vi "Screen_Test.vi"() -> ()   [LabVIEW 2011]
uses:
  030 - EVENTS/EnumFgvEventCommand.ctl
  090 - ERRORS/Ctrls/enumLogAndView.ctl
  SubVis/Ctrls/EnumLockUnlockScreen.ctl
  enumScreen.ctl
  100_PROCESS/SubVis/Enum_HideShow_Process.ctl
  03 - POPUPS/Popup_ShowHideProcess.ctl
  100_PROCESS/SubVis/EnumFgvReferenceProcess.ctl
  100_PROCESS/EnumProcess.ctl
  090 - ERRORS/Ctrls/EnumErrors.ctl
  SubVis/Ctrls/EnumStartStopProgressBar.ctl
  SubVis/Ctrls/EnumEnableDisableClose.ctl
panel:
  out "Process":T1[](array[typedef])
  in  "Window_State":T3(ring)=enum."Standard"
  in  "BoutonSetWindowState":bool
  in  "Hide / Show front panel":T2
  in  "BoutonShowHide":bool
  in  "Bouton menu principal":bool
  in  "Clear message":bool
  in  "Send Error X 100":bool
  in  "Load previous screen":bool
  in  "message":string
  in  "ErrorCode":T4
  in  "Send Error":bool
  in  "Load SCREEN":T5=enum."LOG"
  in  "Close application":bool
  in  "LockUnlock":bool
  in  "Progress bar value":u8(slide) max=100 scale=0.0..100.0
  in  "Automatic progress bar on ?":T6=enum."Stop progress bar"
  in  "Enable close ?":T7
  # "Ecran de test"
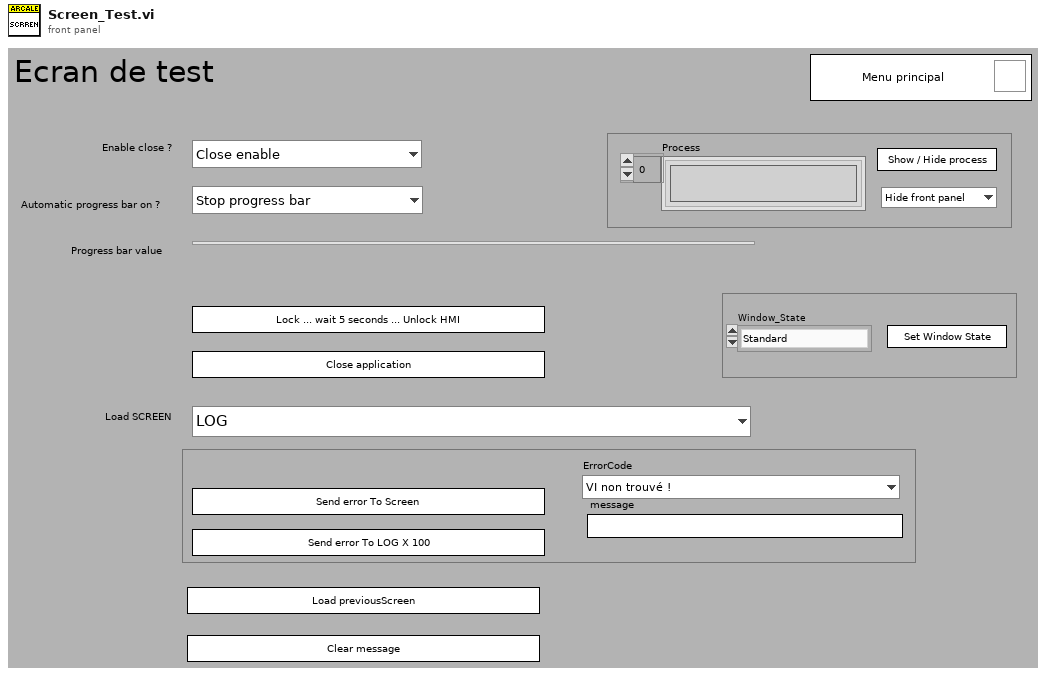
[diagram p1: front panel]
types:
  T1 = typedef "Popup_ShowHideProcess.ctl" = cluster{"Path":path, "VI Name":string, "Hide / Show":T2}
  T2 = typedef "Enum_HideShow_Process.ctl" = enum16{"Hide front panel", "Show front panel"}
  T3 = enum32{"Invalid", "Standard", "Closed", "Hidden", "Minimized", "Maximized"}
  T4 = typedef "EnumErrors.ctl" = enum16{"VI non trouvé !", "Clé non trouvée", "Timeout", "Le VI tourne déjà", "Erreur de séparateur décimal", "Référence non trouvée"}
  T5 = typedef "enumScreen.ctl" = enum16{"Test screen", "Ecran principal", "LOG", "Setup", "Popup : About", "Popup : View last message", "Popup : WebBrowser help", "Traduction", "Popup : DEBUG Process"}
  T6 = typedef "EnumStartStopProgressBar.ctl" = enum16{"Start progress bar", "Stop progress bar"}
  T7 = typedef "EnumEnableDisableClose.ctl" = enum16{"Close enable", "Close disable"}
  T8 = typedef "EnumProcess.ctl" = enum16{"Message handler", "Template"}
  T9 = typedef "EnumFgvReferenceProcess.ctl" = enum16{"Init", "Get", "Add Reference", "Close References"}
  T10 = typedef "enumLogAndView.ctl" = enum16{"Log only", "Log and view"}
  T11 = typedef "EnumFgvEventCommand.ctl" = enum16{"Setup", "Cleanup", "Get"}
  T12 = typedef "EnumLockUnlockScreen.ctl" = enum16{"Lock screen", "Unlock screen"}
  T13 = typedef "ToScreensCommand.ctl" = enum16{"Stop screen", "Stop all screens"}
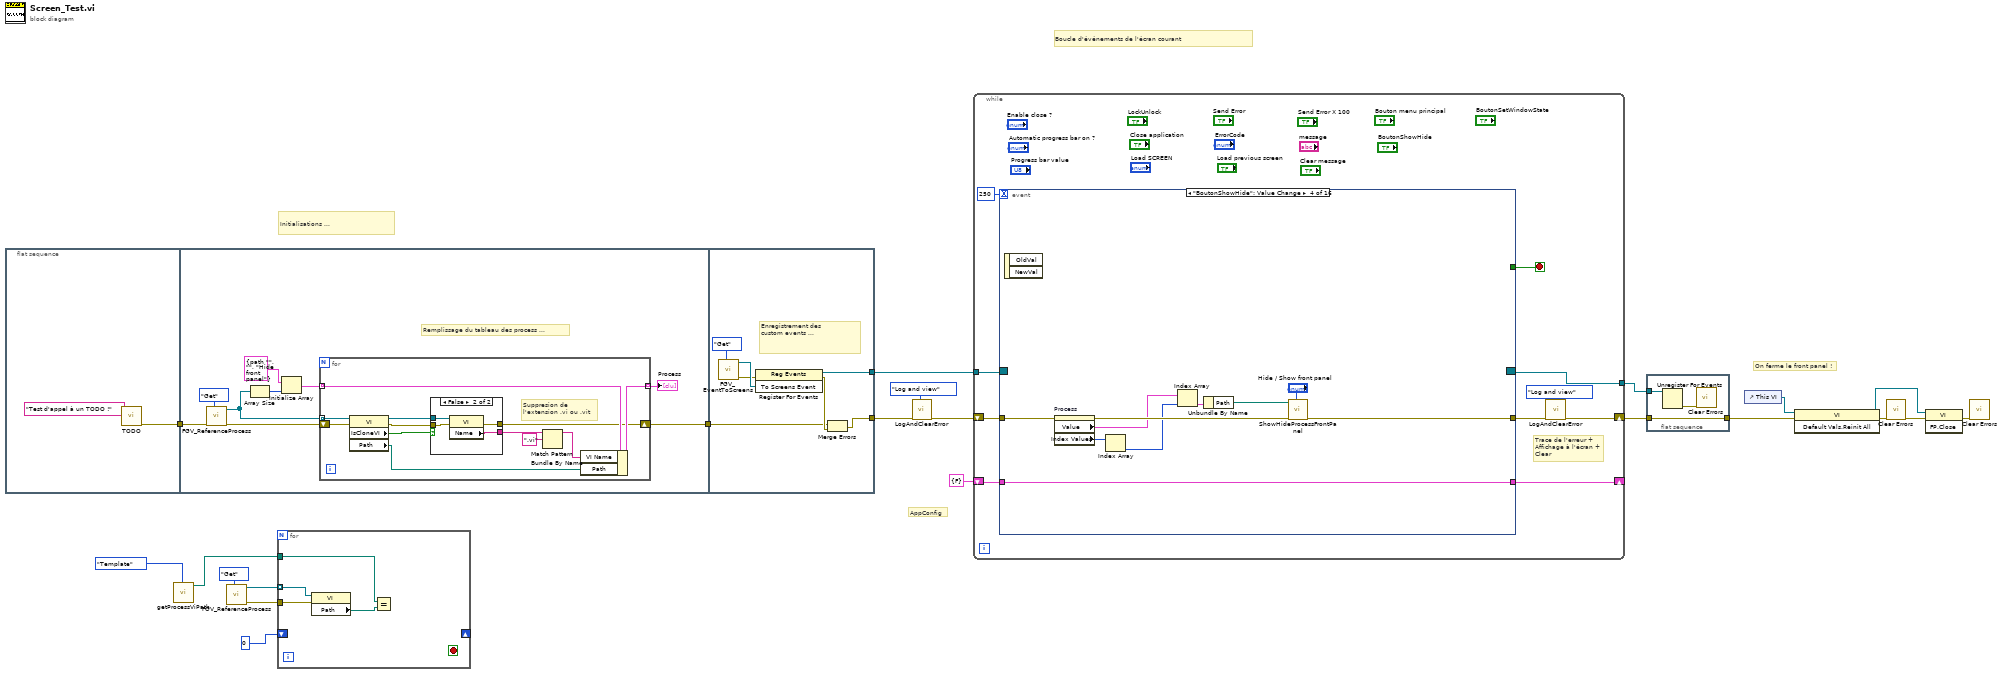
[diagram p0: block diagram]
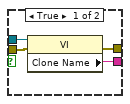
[diagram p2: hidden frame]
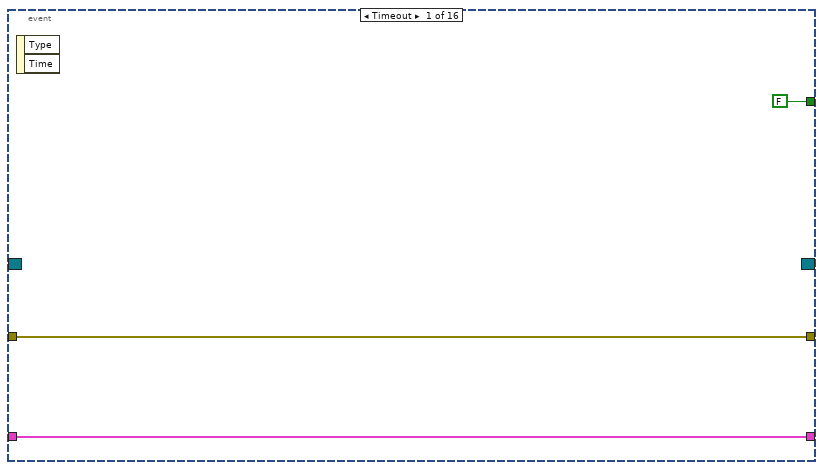
[diagram p3: hidden frame]
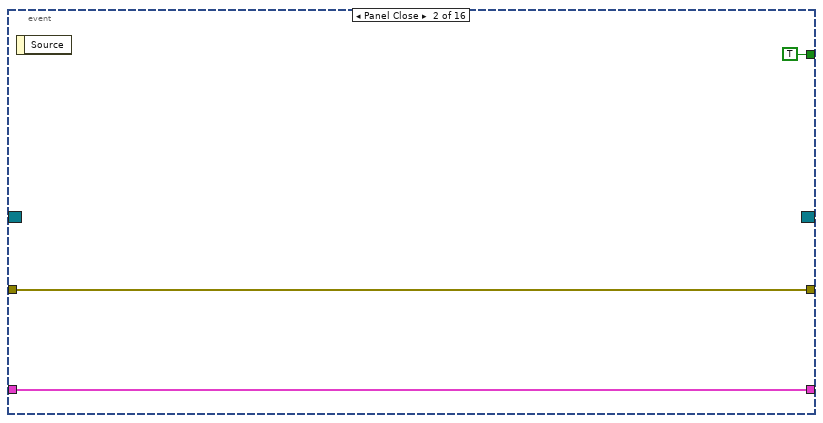
[diagram p4: hidden frame]
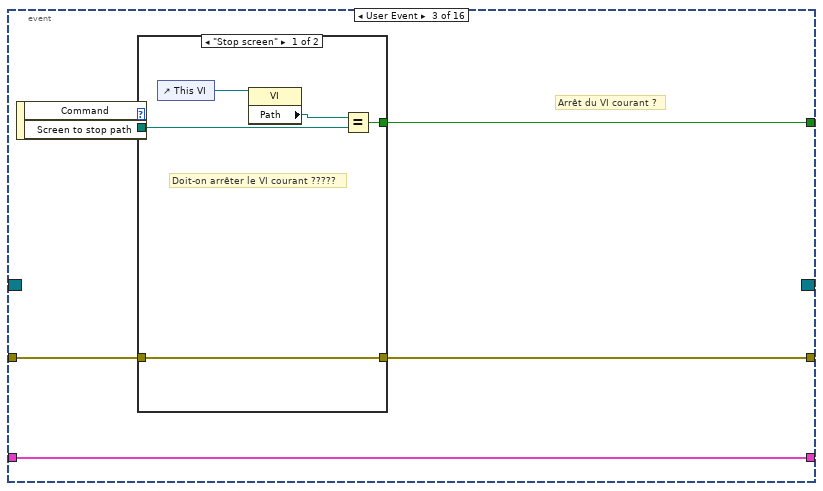
[diagram p5: hidden frame]
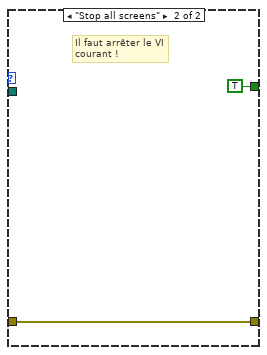
[diagram p6: hidden frame]
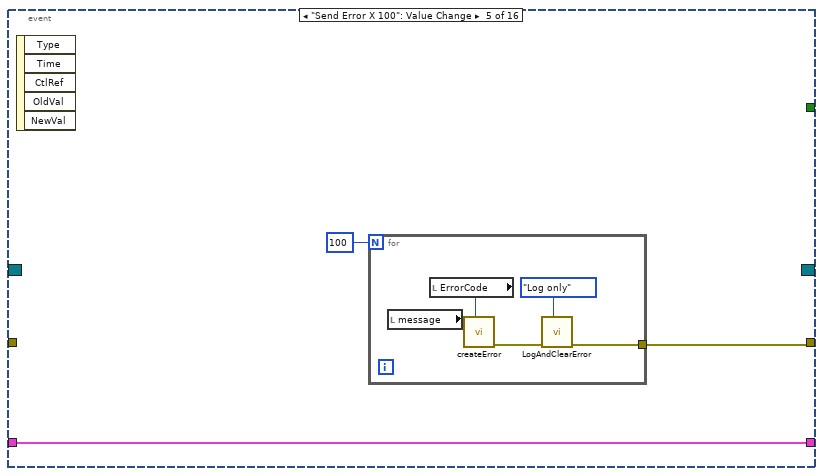
[diagram p7: hidden frame]
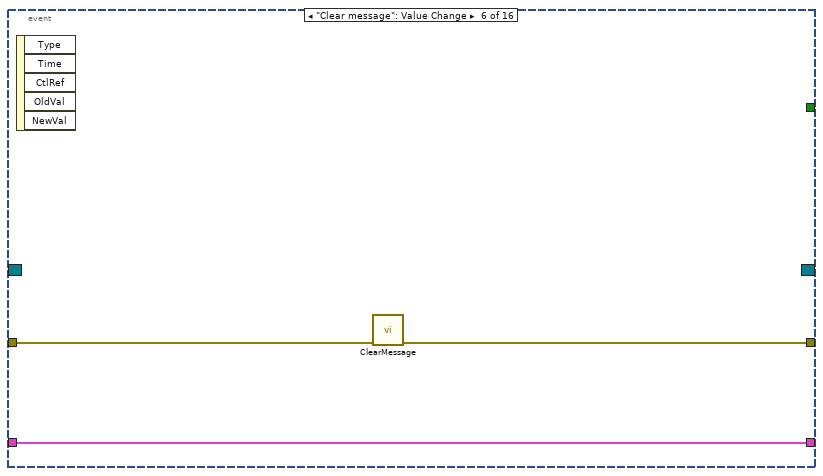
[diagram p8: hidden frame]
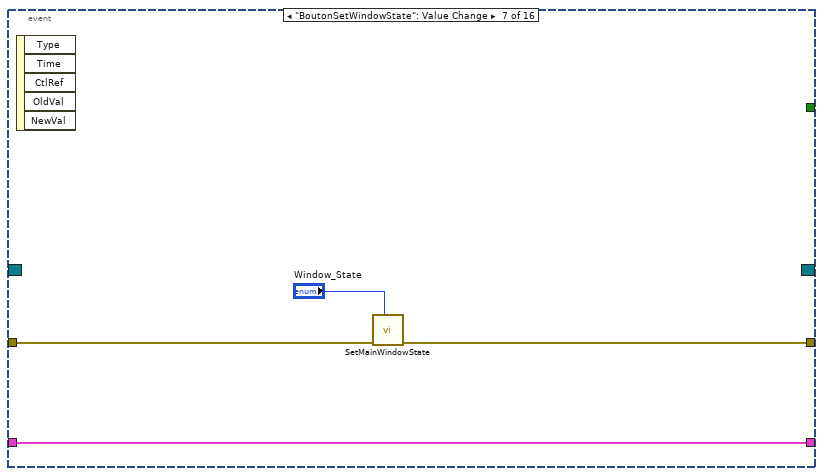
[diagram p9: hidden frame]
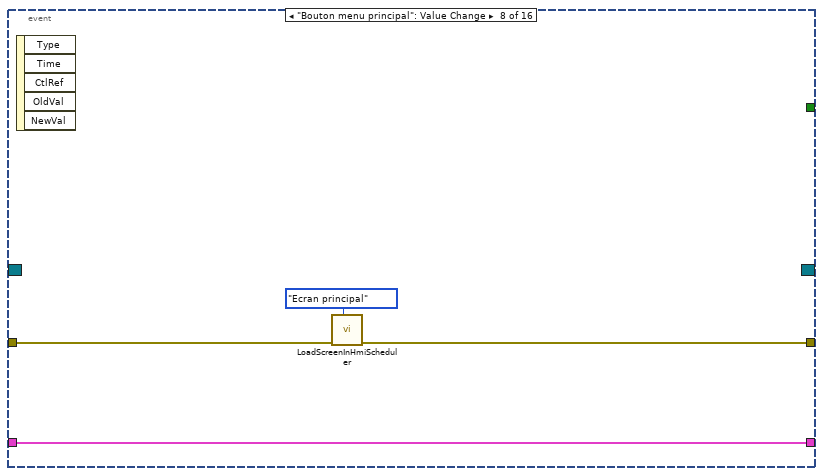
[diagram p10: hidden frame]
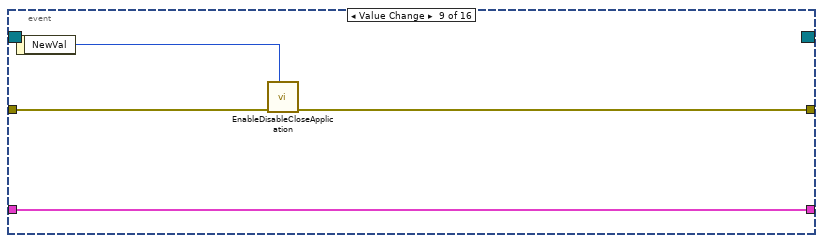
[diagram p11: hidden frame]
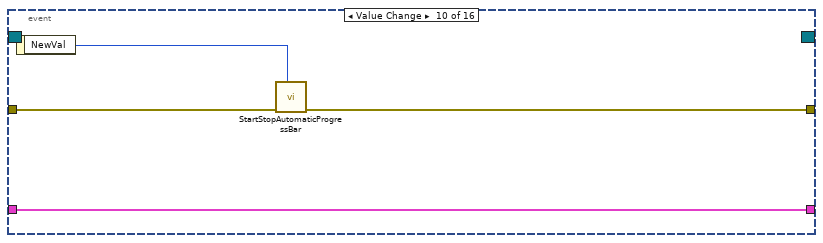
[diagram p12: hidden frame]
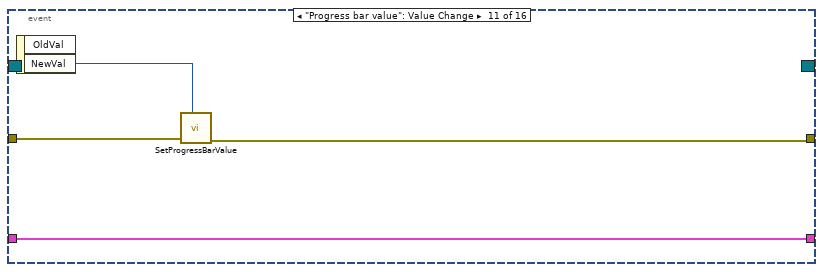
[diagram p13: hidden frame]
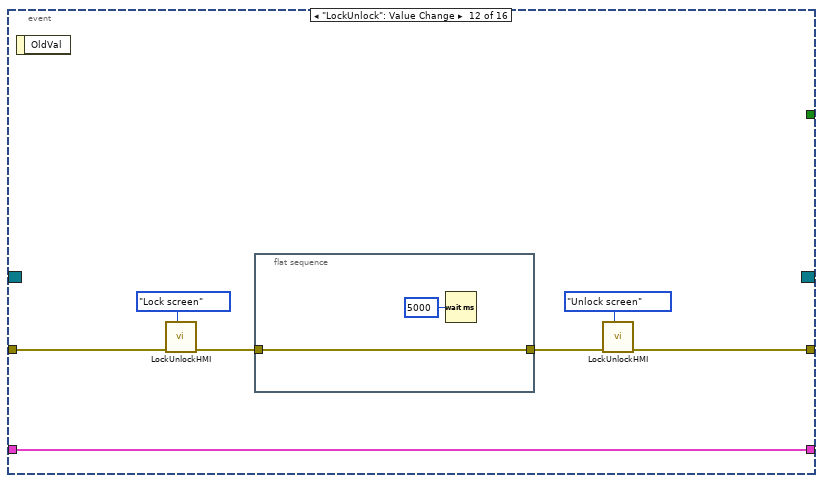
[diagram p14: hidden frame]
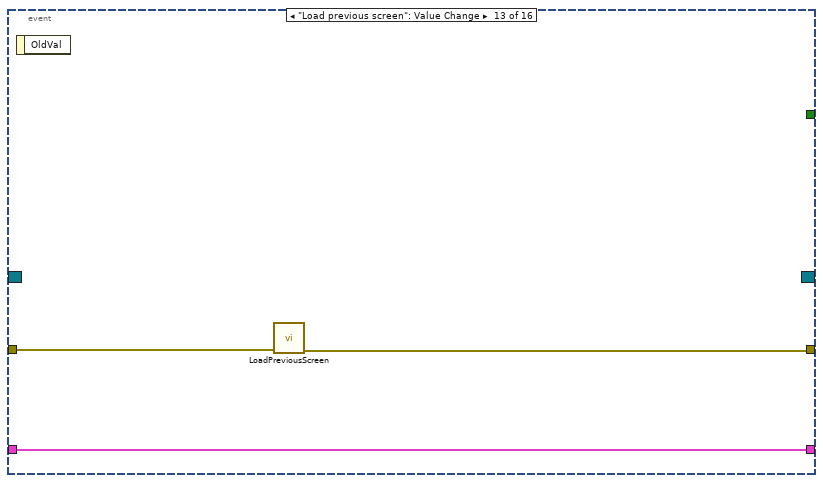
[diagram p15: hidden frame]
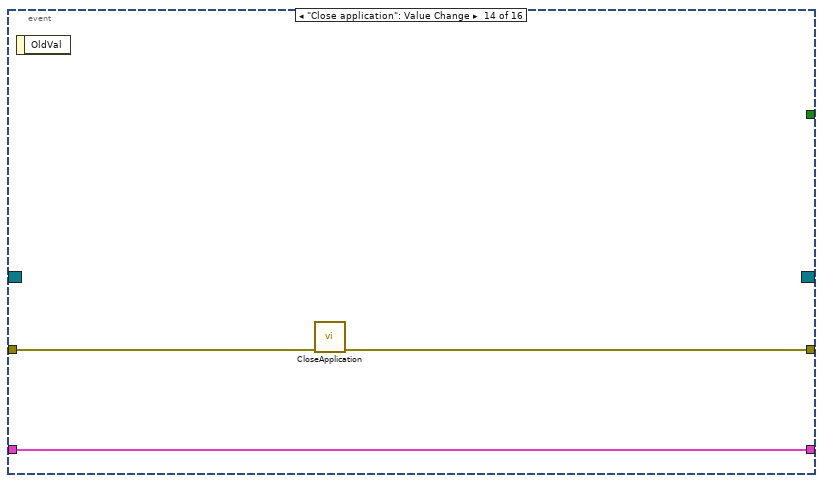
[diagram p16: hidden frame]
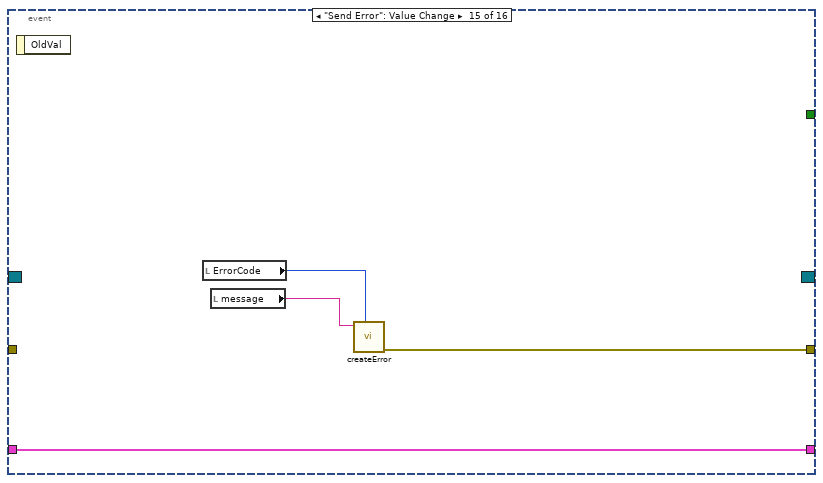
[diagram p17: hidden frame]
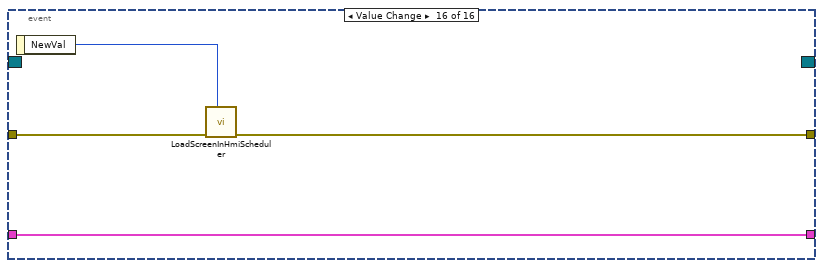
[diagram p18: hidden frame]
diagram:
  # "AppConfig"
  # "Initialisations ..."
  # "On ferme le front panel !"
  # "Boucle d'événements de l'écran courant"
  n1 = flat-sequence {
    tunnel: [w22] -> w8
    tunnel: w8 -> [w27]
    tunnel: [w26] -> w7
    tunnel: w7 -> [w54]
    tunnel: [w55] -> w17
    tunnel: [w53] -> w14
    frame #0 {
      n2 = call "TODO.vi"("Message"="Test d'appel à un TODO !") -> ("error out"=w22:errorcluster)  [unwired: 10 in]
    }
    frame #1 {
      # "Remplissage du tableau des process ..."
      n3 = call "FGV_ReferenceProcess.vi"("Commande"=EnumFgvReferenceProcess."Get", "error in (no error)"=w27) -> ("error out"=w29:errorcluster, "ProcessReferences"=w28:refnum<vi>[])  [unwired: 8 in]
      n4 = Array Size(array=w28) -> (size(s)=w31:i32)
      n5 = Initialize Array(T1 {"Path"=path "", "VI Name"="", "Hide / Show"=enum."Hide front panel"}, w31) -> (w30:T1[])
      n6 = for {
        tunnel: [w44] -> w25 mode=indexing
        tunnel: w28 -> [w41] mode=indexing
        tunnel: w30 -> [w43] mode=indexing
        shift-right: [w36] -> w26
        shift-left: w29 -> [w42]
        # "Suppresion de l'extension .vi ou .vit"
        n7 = property class="VI"(reference=w41, error in=w42) -> (reference out=w38:refnum<vi>, error out=w37:errorcluster, "IsCloneVI"=w39:bool, "Path"=w40:path)
        n8 = case shown="False" w39 {
          tunnel: w38 -> [w48 w52]
          tunnel: w37 -> [w47 w51]
          tunnel: [w46 w50] -> w36
          tunnel: [w45 w49] -> w34
          frame True {
            n9 = property class="VI"(reference=w48, error in=w47) -> (error out=w46:errorcluster, "Clone Name"=w45:string)  [unwired: 1 out]
          }
          frame False {
            n10 = property class="VI"(reference=w52, error in=w51) -> (error out=w50:errorcluster, "Name"=w49:string)  [unwired: 1 out]
          }
        }
        n11 = Match Pattern(string=w34, regular expression=".vi") -> (before substring=w33:string)  [unwired: 1 in, 3 out]
        n12 = Bundle By Name(cluster=w43, "VI Name"=w33, "Path"=w40) -> (w44:T1)
      }
      "Process" <- w25
    }
    frame #2 {
      # "Enregistrement des\ncustom events ..."
      n13 = call "FGV_EventToScreens.vi"("Command"=EnumFgvEventCommand."Get") -> ("error out"=w57:errorcluster, "To Screens Event"=w58:refnum<user-event>)  [unwired: 9 in]
      n14 = register-events(error in=w57, w58) -> (reference out=w55:refnum<event-registration>, error out=w59:errorcluster)  [unwired: 1 in]
      n15 = Merge Errors(w54, w59) -> (w53:errorcluster)
    }
  }
  n16 = call "getProcessViPath.vi"("Enum Screen"=EnumProcess."Template" ("Process")) -> ("Path"=w2:path)  [unwired: 9 in, 1 out]
  n17 = call "FGV_ReferenceProcess.vi"("Commande"=EnumFgvReferenceProcess."Get") -> ("error out"=w4:errorcluster, "ProcessReferences"=w5:refnum<vi>[])  [unwired: 9 in]
  n18 = for {
    tunnel: w5 -> [w63] mode=indexing
    tunnel: w4 -> [w62]
    tunnel: w2 -> [w60]
    shift-right: _ -> [_]
    shift-left: 0 -> [_]
    stop <- _ stop-if-true
    n19 = property class="VI"(reference=w63, error in=w62) -> ("Path"=w61:path)  [unwired: 2 out]
    n20 = Equal?(x=w60, y=w61) -> ()  [unwired: 1 out]
  }
  n21 = call "LogAndClearError.vi"("Log and view ?"=enumLogAndView."Log and view", "error in (no error)"=w14) -> ("error out"=w15:errorcluster)  [unwired: 9 in]
  n22 = while {
    tunnel: w17 -> [w73]
    shift-right: [w67] -> w20
    shift-left: w15 -> [w72]
    tunnel: [w71] -> w21
    shift-right: [w68] -> _
    shift-left: cluster{"Boolean":bool} {"Boolean"=FALSE} ("appContext") -> [w69]
    stop <- w70 stop-if-true
    # "Trace de l'erreur +\nAffichage à l'écran +\nClear"
    n23 = event shown="[3] \"BoutonShowHide\": Value Change" {
      selector: w73 -> [_ _ _ _ _ _ _ _ _ _ _ _ _ _ _ _]
      dyn-events: [_ _ _ _ _ _ _ _ _ _ _ _ _ _ _ _] -> w71
      timeout: 250 -> [_ _ _ _ _ _ _ _ _ _ _ _ _ _ _ _]
      tunnel: w72 -> [w76 w79 w84 w99 _ w113 w117 w120 w124 w129 w133 w140 w145 w148 _ w156]
      tunnel: [w76 w79 w83 w102 w105 w112 w116 w119 w123 w128 w132 w136 w144 w147 w150 w154] -> w66
      tunnel: [FALSE TRUE w81 _ _ _ _ _ _ _ _ _ _ _ _ _] -> w70
      tunnel: w69 -> [w74 w78 w80 w101 w103 w111 w115 w121 w125 w127 w131 w139 w143 w146 w152 w153]
      tunnel: [w74 w78 w80 w101 w103 w111 w115 w121 w125 w127 w131 w139 w143 w146 w152 w153] -> w68
      event Timeout {
        n24 = event-data() -> ()  [unwired: 1 in, 2 out]
      }
      event Panel Close {
        n25 = event-data() -> ()  [unwired: 1 in, 1 out]
      }
      event User Event {
        # "Arrêt du VI courant ?"
        n26 = event-data() -> ("Command"=w85:T13, "Screen to stop path"=w82:path)  [unwired: 1 in]
        n27 = case shown="\"Stop screen\"" w85 {
          tunnel: w84 -> [w90 w91]
          tunnel: [w90 w91] -> w83
          tunnel: w82 -> [w87 _]
          tunnel: [w86 TRUE] -> w81
          frame "Stop screen" {
            # "Doit-on arrêter le VI courant ?????"
            n28 = control-ref of="This VI"() -> (w89:refnum<vi>)
            n29 = property class="VI"(reference=w89) -> ("Path"=w88:path)  [unwired: 1 in, 2 out]
            n30 = Equal?(x=w88, y=w87) -> (x = y?=w86:bool)
          }
          frame "Stop all screens" {
            # "Il faut arrêter le VI\ncourant !"
          }
        }
      }
      event "BoutonShowHide": Value Change {
        n31 = event-data() -> ()  [unwired: 1 in, 2 out]
        n32 = property on="Process" class="Arr (strict)"(error in=w99) -> (error out=w98:errorcluster, "Value"=w97:T1[], "Index Values"=w96:u32[])  [unwired: 1 in, 1 out]
        n33 = Index Array(array=w96) -> (element=w95:u32)  [unwired: 1 in]
        n34 = Index Array(array=w97, index=w95) -> (element=w94:T1)
        n35 = Unbundle By Name(w94) -> ("Path"=w93:path)
        n36 = call "ShowHideProcessFrontPanel.vi"("Hide / Show front panel"="Hide / Show front panel", "error in (no error)"=w98, "Process path"=w93) -> ("error out"=w102:errorcluster)  [unwired: 8 in]
      }
      event "Send Error X 100": Value Change {
        n37 = event-data() -> ()  [unwired: 1 in, 5 out]
        n38 = for {
          N: 100 -> [_]
          tunnel: [w107] -> w105
          n39 = local read "message"() -> (w109:string)
          n40 = local read "ErrorCode"() -> (w110:T4)
          n41 = call "createError.vi"("ErrorCode"=w110, "message"=w109) -> ("error out"=w108:errorcluster)  [unwired: 9 in]
          n42 = call "LogAndClearError.vi"("Log and view ?"=enumLogAndView."Log only", "error in (no error)"=w108) -> ("error out"=w107:errorcluster)  [unwired: 9 in]
        }
      }
      event "Clear message": Value Change {
        n43 = event-data() -> ()  [unwired: 1 in, 5 out]
        n44 = call "ClearMessage.vi"("error in (no error)"=w113) -> ("error out"=w112:errorcluster)  [unwired: 10 in]
      }
      event "BoutonSetWindowState": Value Change {
        n45 = event-data() -> ()  [unwired: 1 in, 5 out]
        n46 = call "SetMainWindowState.vi"("Window_State"="Window_State", "error in (no error)"=w117) -> ("error out"=w116:errorcluster)  [unwired: 9 in]
      }
      event "Bouton menu principal": Value Change {
        n47 = event-data() -> ()  [unwired: 1 in, 5 out]
        n48 = call "LoadScreenInHmiScheduler.vi"("Enum Screen"=enumScreen."Ecran principal", "error in (no error)"=w120) -> ("error out"=w119:errorcluster)  [unwired: 9 in]
      }
      event Value Change {
        n49 = event-data() -> ("NewVal"=w122:T7)  [unwired: 1 in]
        n50 = call "EnableDisableCloseApplication.vi"("Close enable/disable"=w122, "error in (no error)"=w124) -> ("error out"=w123:errorcluster)  [unwired: 9 in]
      }
      event Value Change {
        n51 = event-data() -> ("NewVal"=w126:T6)  [unwired: 1 in]
        n52 = call "StartStopAutomaticProgressBar.vi"("Start / Stop ?"=w126, "error in (no error)"=w129) -> ("error out"=w128:errorcluster)  [unwired: 9 in]
      }
      event "Progress bar value": Value Change {
        n53 = event-data() -> ("NewVal"=w130:u8)  [unwired: 1 in, 1 out]
        n54 = call "SetProgressBarValue.vi"("Progress bar value"=w130, "error in (no error)"=w133) -> ("error out"=w132:errorcluster)  [unwired: 9 in]
      }
      event "LockUnlock": Value Change {
        n55 = event-data() -> ()  [unwired: 1 in, 1 out]
        n56 = call "LockUnlockHMI.vi"("Lock / unlock screen ?"=EnumLockUnlockScreen."Lock screen", "error in (no error)"=w140) -> ("error out"=w138:errorcluster)  [unwired: 9 in]
        n57 = flat-sequence {
          tunnel: w138 -> [w142]
          tunnel: [w142] -> w137
          frame #0 {
            n58 = Wait (ms)(milliseconds to wait=u32 5000) -> ()  [unwired: 1 out]
          }
        }
        n59 = call "LockUnlockHMI.vi"("Lock / unlock screen ?"=EnumLockUnlockScreen."Unlock screen", "error in (no error)"=w137) -> ("error out"=w136:errorcluster)  [unwired: 9 in]
      }
      event "Load previous screen": Value Change {
        n60 = event-data() -> ()  [unwired: 1 in, 1 out]
        n61 = call "LoadPreviousScreen.vi"("error in (no error)"=w145) -> ("error out"=w144:errorcluster)  [unwired: 10 in]
      }
      event "Close application": Value Change {
        n62 = event-data() -> ()  [unwired: 1 in, 1 out]
        n63 = call "CloseApplication.vi"("error in (no error)"=w148) -> ("error out"=w147:errorcluster)  [unwired: 10 in]
      }
      event "Send Error": Value Change {
        n64 = event-data() -> ()  [unwired: 1 in, 1 out]
        n65 = local read "ErrorCode"() -> (w151:T4)
        n66 = local read "message"() -> (w149:string)
        n67 = call "createError.vi"("ErrorCode"=w151, "message"=w149) -> ("error out"=w150:errorcluster)  [unwired: 9 in]
      }
      event Value Change {
        n68 = event-data() -> ("NewVal"=w155:T5)  [unwired: 1 in]
        n69 = call "LoadScreenInHmiScheduler.vi"("Enum Screen"=w155, "error in (no error)"=w156) -> ("error out"=w154:errorcluster)  [unwired: 9 in]
      }
    }
    n70 = call "LogAndClearError.vi"("Log and view ?"=enumLogAndView."Log and view", "error in (no error)"=w66) -> ("error out"=w67:errorcluster)  [unwired: 9 in]
  }
  n71 = flat-sequence {
    tunnel: w21 -> [w159]
    tunnel: w20 -> [w157]
    tunnel: [w157] -> w12
    frame #0 {
      n72 = Unregister For Events(event registration refnum=w159) -> (error out=w158:errorcluster)  [unwired: 1 in]
      n73 = call <vilib>:"Clear Errors.vi"("error in (no error)"=w158) -> ()  [unwired: 6 in, 1 out]
    }
  }
  n74 = control-ref of="This VI"() -> (w11:refnum<vi>)
  n75 = invoke class="VI" method="Default Vals.Reinit All"(reference=w11, error in=w12) -> (reference out=w10:refnum<vi>, error out=w13:errorcluster)  [unwired: 1 in, 1 out]
  n76 = call <vilib>:"Clear Errors.vi"("error in (no error)"=w13) -> ("error out"=w9:errorcluster)  [unwired: 6 in]
  n77 = invoke class="VI" method="FP.Close"(reference=w10, error in=w9) -> (error out=w19:errorcluster)  [unwired: 1 in, 2 out]
  n78 = call <vilib>:"Clear Errors.vi"("error in (no error)"=w19) -> ()  [unwired: 6 in, 1 out]
